vi "Ctor.vi"(8 "error in (no error)":errorcluster, 11 "DeviceDetailPanel in":refnum<class "DeviceDetailPanel.lvclass">) -> (0 "error out":errorcluster, 3 "DeviceDetailPanel out":refnum<class "DeviceDetailPanel.lvclass">)   [LabVIEW 2020, in "PicoG-App.lvlib" / "DeviceDetailPanel.lvclass"]
uses:
  DeviceDetailPanel.lvclass
  Ref Data.ctl
  Device/Device.lvclass
  DeviceDetailPanel.lvclass/DeviceDetailPanel.ctl
  <vilib>/IlluminatedG/IG OOPanel/OOPanel/Panel/Panel.lvclass
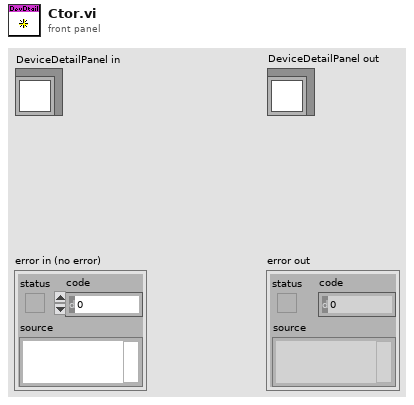
[diagram p1: front panel]
types:
  T1 = typedef "PicoG-App.lvlib/DeviceDetailPanel.lvclass/Ref Data.ctl" = cluster{"Device":refnum<class "Device.lvclass">}
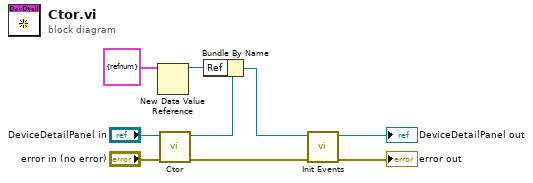
[diagram p0: block diagram]
diagram:
  n1 = New Data Value Reference(data value=T1 {"Device"=refnum} ("Ref Data")) -> (data value reference=w5:refnum<data-value>)  [unwired: 1 in, 1 out]
  n2 = call-parent "Ctor.vi"("error in (no error)"="error in (no error)", "Panel in"="DeviceDetailPanel in") -> ("error out"=w1:errorcluster, "Panel out"=w7:refnum<class "DeviceDetailPanel.lvclass">)  [unwired: 8 in]
  n3 = Bundle By Name(cluster=w7, "Ref"=w5) -> (w2:refnum<class "DeviceDetailPanel.lvclass">)
  n4 = call "Init Events.vi"("error in (no error)"=w1, "DeviceDetailPanel in"=w2) -> ("error out"=→"error out":errorcluster, "DeviceDetailPanel out"=→"DeviceDetailPanel out":refnum<class "DeviceDetailPanel.lvclass">)  [unwired: 8 in]
